vi "Apply Impact Force.vi"(10 "force":dbl, 11 "Poundable in":refnum<class "Poundable.lvclass">) -> (3 "Poundable out":refnum<class "Poundable.lvclass">)   [LabVIEW 2023, in "Poundable.lvclass"]
uses:
  Poundable.lvclass
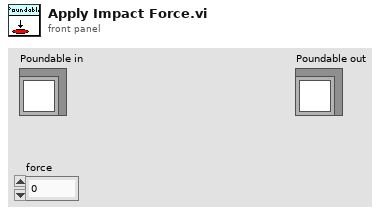
[diagram p1: front panel]
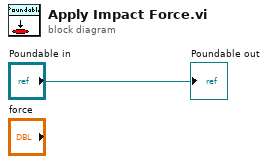
[diagram p0: block diagram]
diagram:
  "Poundable out" <- "Poundable in"
